vi "receive message.vi"(8 "error in (no error)":errorcluster, 11 "Communication Manager in":refnum<class "Communication Manager.lvclass">) -> (0 "error out":errorcluster, 3 "Communication Manager out":refnum<class "Communication Manager.lvclass">)   [LabVIEW 2018, in "Communication Manager.lvclass"]
uses:
  Communication Manager.lvclass
  Communication Manager.lvclass/Communication Manager.ctl
  Socket/Socket.lvclass
  RxTx/RxTx.lvclass
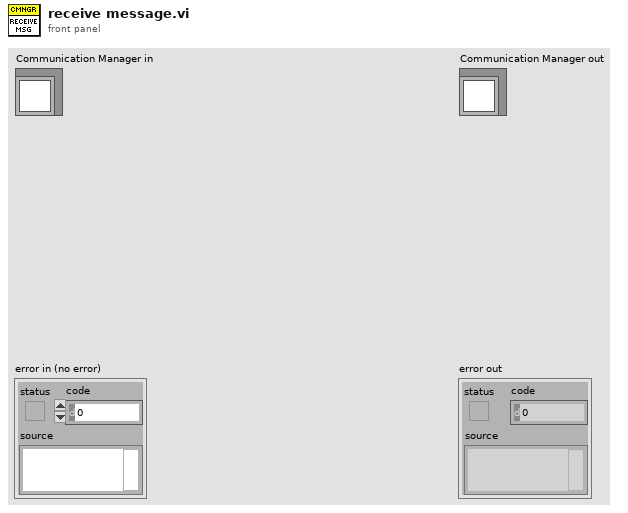
[diagram p1: front panel]
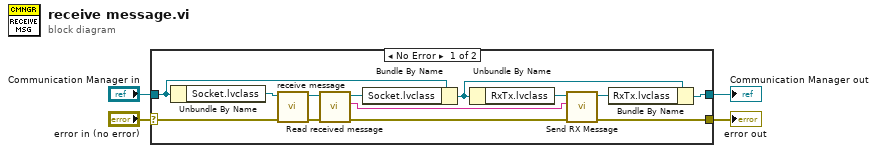
[diagram p0: block diagram]
diagram:
  n1 = case shown="No Error" "error in (no error)" {
    selector: "error in (no error)" -> [w16 w19]
    tunnel: [w6 w19] -> w3
    tunnel: [w5 w18] -> w1
    tunnel: "Communication Manager in" -> [w15 w18]
    frame No Error {
      n2 = Unbundle By Name(w15) -> ("Socket.lvclass"=w17:refnum<class "Socket.lvclass">)
      n3 = call-dynamic "receive message.vi"("error in (no error)"=w16, "Socket in"=w17) -> ("error out"=w13:errorcluster, "Socket out"=w14:refnum<class "Socket.lvclass">)  [unwired: 8 in]
      n4 = call-dynamic "Read received message.vi"("error in (no error)"=w13, "Socket in"=w14) -> ("error out"=w10:errorcluster, "received message"=w9:string, "Socket out"=w12:refnum<class "Socket.lvclass">)  [unwired: 7 in]
      n5 = Bundle By Name(cluster=w15, "Socket.lvclass"=w12) -> (w8:refnum<class "Communication Manager.lvclass">)
      n6 = Unbundle By Name(w8) -> ("RxTx.lvclass"=w11:refnum<class "RxTx.lvclass">)
      n7 = call "Send RX Message.vi"("error in (no error)"=w10, "message"=w9, "RxTx in"=w11) -> ("error out"=w6:errorcluster, "RxTx out"=w7:refnum<class "RxTx.lvclass">)  [unwired: 7 in]
      n8 = Bundle By Name(cluster=w8, "RxTx.lvclass"=w7) -> (w5:refnum<class "Communication Manager.lvclass">)
    }
    frame Error {
    }
  }
  "error out" <- w3
  "Communication Manager out" <- w1
